vi "RSVNA save s-parameters.vi"() -> ()   [LabVIEW 2020]
uses:
  <instrlib>/Rohde&Schwarz Vector Network Analyzer/Rohde&Schwarz Vector Network Analyzer.lvlib
  Instruments/Vector Network Analyzer/Controls/Sparameter cluster.ctl
  Instruments/Vector Network Analyzer/Vector Network Analyzer.lvclass
panel:
  in  "File Path":path
  in  "Note":string
  out "Array":i32[](array[numeric])
  out "array":string[](array[string])
  out "Trace Data":cdb[][](array[numeric])
  in  "Channel (1)":i32=1
  in  "Number of Logical Ports (1)":i32=1
  in  "Logical Ports":i32[](array[numeric])
  in  "error in (no error)":errorcluster
  in  "Reset (T: Reset)":bool=TRUE
  in  "ID Query (T: Check)":bool=TRUE
  in  "VISA resource name":refnum<visa-resource-name>
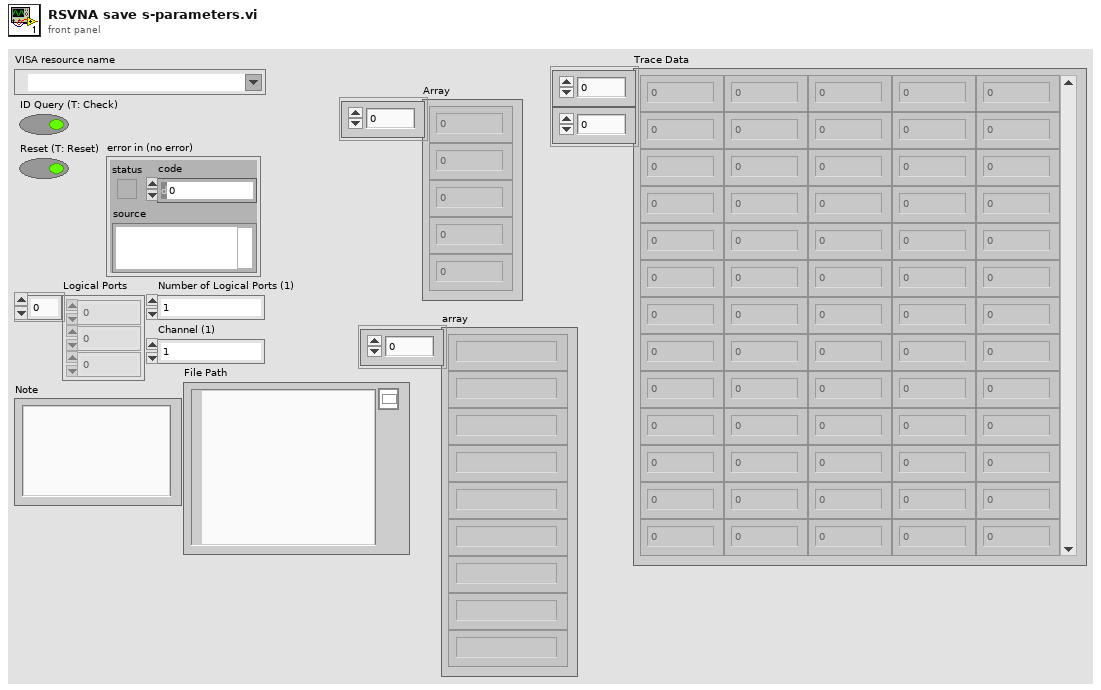
[diagram p1: front panel]
types:
  T1 = typedef "Vector Network Analyzer.lvclass/Sparameter cluster.ctl" = cluster{"Frequency":dbl, "S Parameters":cdb[]}
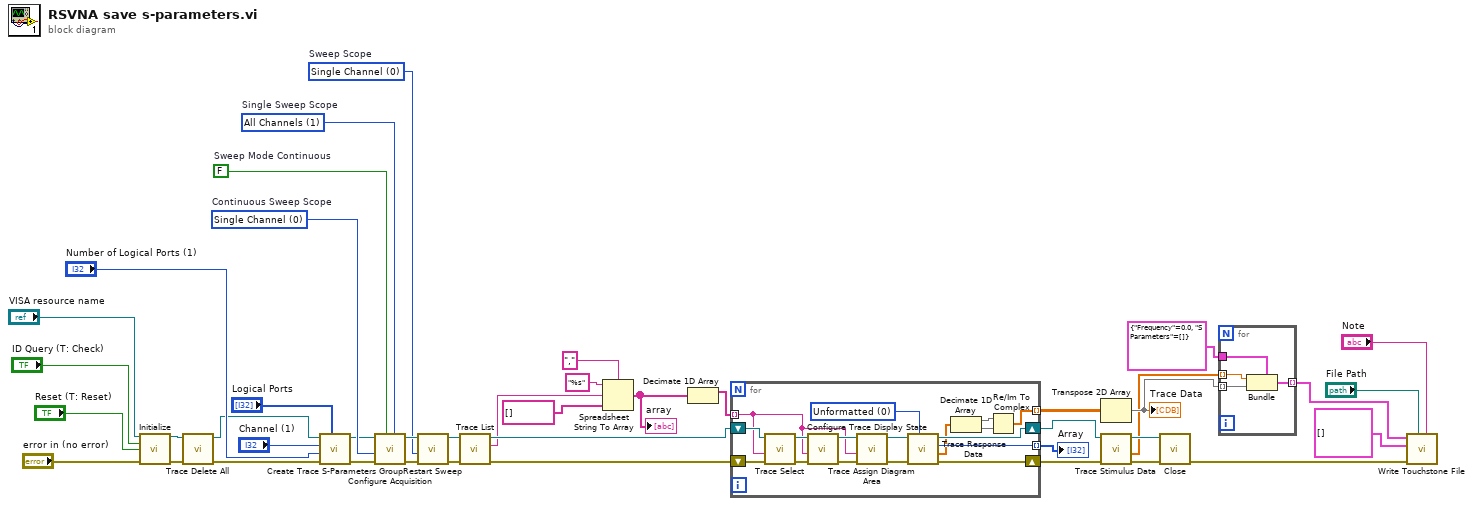
[diagram p0: block diagram]
diagram:
  w17 = 0 items=["Single Channel", "All Channels"]  # Sweep Scope
  w20 = 0 items=["Single Channel", "All Channels"]  # Continuous Sweep Scope
  w21 = FALSE  # Sweep Mode Continuous
  w22 = 1 items=["Single Channel", "All Channels"]  # Single Sweep Scope
  n1 = call <instrlib>:"Initialize.vi"("VISA resource name"="VISA resource name", "ID Query (T: Check)"="ID Query (T: Check)", "Reset (T: Reset)"="Reset (T: Reset)", "error in (no error)"="error in (no error)") -> ("VISA resource name out"=w27:refnum<visa-resource-name>, "error out"=w26:errorcluster)  [unwired: 10 in]
  n2 = call <instrlib>:"Trace Delete All.vi"("error in (no error)"=w26, "VISA resource name"=w27) -> ("error out"=w25:errorcluster, "VISA resource name out"=w24:refnum<visa-resource-name>)  [unwired: 8 in]
  n3 = call <instrlib>:"Create Trace S-Parameters Group.vi"("Logical Ports"="Logical Ports", "error in (no error)"=w25, "Number of Logical Ports (1)"="Number of Logical Ports (1)", "Channel (1)"="Channel (1)", "VISA resource name"=w24) -> ("error out"=w15:errorcluster, "VISA resource name out"=w16:refnum<visa-resource-name>)  [unwired: 5 in]
  n4 = call <instrlib>:"Configure Acquisition.vi"("Single Sweep Scope (All Channels)"=w22, "Sweep Mode Continuous (F)"=w21, "error in (no error)"=w15, "Continuous Sweep Scope (All Channels)"=w20, "VISA resource name"=w16) -> ("error out"=w19:errorcluster, "VISA resource name out"=w18:refnum<visa-resource-name>)  [unwired: 5 in]
  n5 = call <instrlib>:"Restart Sweep.vi"("error in (no error)"=w19, "Sweep Scope (All Channels)"=w17, "VISA resource name"=w18) -> ("error out"=w14:errorcluster, "VISA resource name out"=w13:refnum<visa-resource-name>)  [unwired: 7 in]
  n6 = call <instrlib>:"Trace List.vi"("error in (no error)"=w14, "VISA resource name"=w13) -> ("error out"=w35:errorcluster, "Catalog"=w34:string, "VISA resource name out"=w36:refnum<visa-resource-name>)  [unwired: 7 in]
  n7 = Spreadsheet String To Array(delimiter (Tab)=",", format string="%s", spreadsheet string=w34, array type (2D Dbl)=string[] []) -> (array=w30:string[])
  "array" <- w30
  n8 = Decimate 1D Array(w30) -> (w29:string[])  [unwired: 1 out]
  n9 = for {
    shift-right: [w58] -> w6
    shift-left: w36 -> [w60]
    shift-right: [w57] -> w7
    shift-left: w35 -> [w59]
    tunnel: w29 -> [w49] mode=indexing
    tunnel: [w45] -> w28 mode=indexing
    tunnel: [w56] -> w23 mode=indexing
    w44 = 0 items=["Unformatted", "Formatted", "Unformatted With Trace Mathematics"] ("Data Format (Unformatted)")
    n10 = call <instrlib>:"Trace Select.vi"("error in (no error)"=w59, "Trace Name (\"Trc1\")"=w49, "VISA resource name"=w60) -> ("error out"=w55:errorcluster, "VISA resource name out"=w54:refnum<visa-resource-name>)  [unwired: 7 in]
    n11 = call <instrlib>:"Configure Trace Display State.vi"("error in (no error)"=w55, "Single Trace Name (\"Trc1\")"=w49, "VISA resource name"=w54) -> ("error out"=w52:errorcluster, "VISA resource name out"=w53:refnum<visa-resource-name>)  [unwired: 7 in]
    n12 = call <instrlib>:"Trace Assign Diagram Area.vi"("error in (no error)"=w52, "Trace Name (\"Ch1Trc1\")"=w49, "VISA resource name"=w53) -> ("error out"=w50:errorcluster, "VISA resource name out"=w51:refnum<visa-resource-name>)  [unwired: 7 in]
    n13 = call <instrlib>:"Trace Response Data.vi"("Data Format (Unformatted)"=w44, "error in (no error)"=w50, "VISA resource name"=w51) -> ("error out"=w57:errorcluster, "Trace Data"=w46:dbl[], "No of Values"=w56:i32, "VISA resource name out"=w58:refnum<visa-resource-name>)  [unwired: 5 in]
    n14 = Decimate 1D Array(w46) -> (w48:dbl[], w47:dbl[])
    n15 = Re/Im To Complex(1:w47, 2:w48) -> (0:w45:cdb[])
  }
  "Array" <- w23
  n16 = Transpose 2D Array(2D array=w28) -> (transposed array=w8:cdb[][])
  "Trace Data" <- w8
  n17 = call <instrlib>:"Trace Stimulus Data.vi"("error in (no error)"=w7, "VISA resource name"=w6) -> ("error out"=w5:errorcluster, "Trace Data"=w3:dbl[], "VISA resource name out"=w4:refnum<visa-resource-name>)  [unwired: 6 in, 1 out]
  n18 = call <instrlib>:"Close.vi"("error in (no error)"=w5, "VISA resource name"=w4) -> ("error out"=w9:errorcluster)  [unwired: 9 in]
  n19 = for {
    tunnel: w8 -> [w62] mode=indexing
    tunnel: w3 -> [w63] mode=indexing
    tunnel: T1 {"Frequency"=0.0, "S Parameters"=[]} ("S Parameters") -> [w64]
    tunnel: [w61] -> w1 mode=indexing
    n20 = Bundle(cluster=w64, "Frequency"=w63, "S Parameters"=w62) -> (w61:T1)
  }
  n21 = call "Write Touchstone File.vi"("Note"="Note", "File Path"="File Path", "Error In"=w9, "Parameters"=cluster{"Name":string, "Value":string}[] [], "Sparameters"=w1) -> ()  [unwired: 6 in, 1 out]
